vi "Telescope Debug Message.vi"(8 "error in (no error)":errorcluster, 9 "Message":string, 10 "Topic":string, 11 "LDT Telescope in":refnum<class "LDT Telescope.lvclass">) -> (0 "error out":errorcluster, 3 "LDT Telescope out":refnum<class "LDT Telescope.lvclass">)   [LabVIEW 2022 SP3, in "LDT Telescope.lvclass"]
uses:
  LDT Telescope.lvclass
  LDT Telescope.lvclass/LDT Telescope.ctl
  Telescope.lvclass
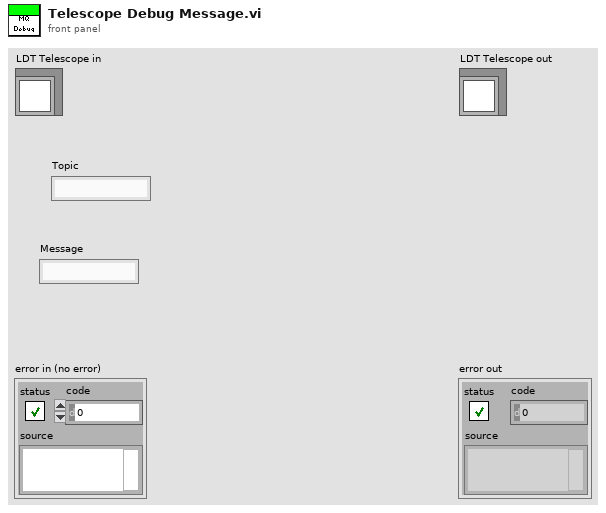
[diagram p1: front panel]
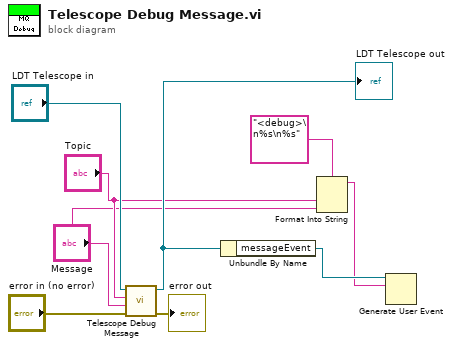
[diagram p0: block diagram]
diagram:
  n1 = call-parent "Telescope Debug Message.vi"("error in (no error)"="error in (no error)", "Message"="Message", "Topic"="Topic", "Telescope in"="LDT Telescope in") -> ("error out"=→"error out":errorcluster, "Telescope out"=w6:refnum<class "LDT Telescope.lvclass">)  [unwired: 6 in]
  "LDT Telescope out" <- w6
  n2 = Unbundle By Name(w6) -> ("messageEvent"=w5:refnum<user-event>)
  n3 = Format Into String(format string="<debug>\n%s\n%s", "Topic", "Message") -> (resulting string=w1:string)  [unwired: 2 in, 1 out]
  n4 = Generate User Event(user event=w5, event data cluster=w1) -> ()  [unwired: 2 in, 2 out]
